vi "Destroy.vi"(8 "error in (no error)":errorcluster, 11 "ServiceName Template in":refnum<class "ServiceName Template.lvclass">) -> (0 "error out":errorcluster, 3 "ServiceName Template out":refnum<class "ServiceName Template.lvclass">)   [LabVIEW 2024, in "ServiceName Template.lvclass"]
uses:
  ServiceName Template.lvclass
  ServiceName Template.lvclass/ServiceName Template.ctl
  gRPC lv Servicer/ServiceBase/ServiceBase.lvclass
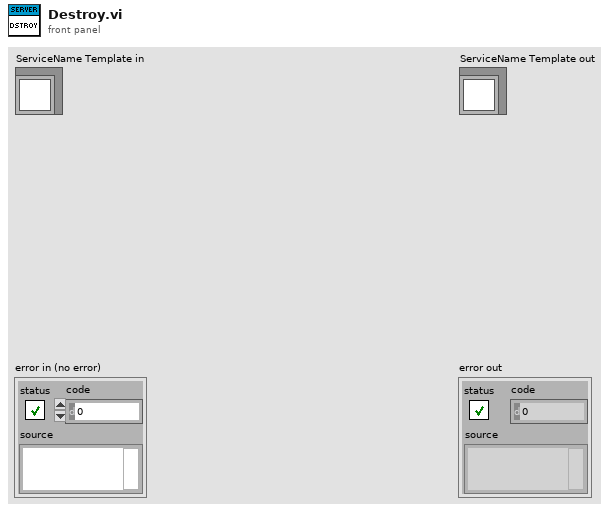
[diagram p1: front panel]
types:
  T1 = typedef "ServiceName Template.lvclass/Server gRPC UEs.ctl" = cluster{"package_service_method":refnum<user-event>}
  T2 = typedef "ServiceName Template.lvclass/Server Internal UEs.ctl" = cluster{"package_service_method Internal UE":refnum<user-event>}
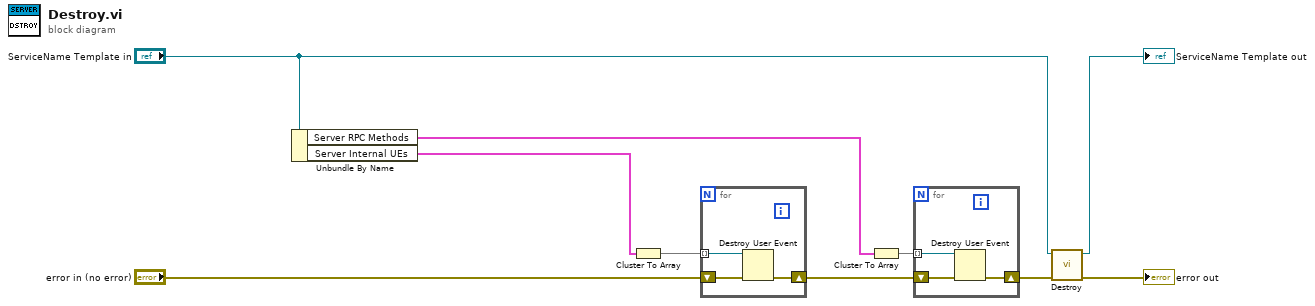
[diagram p0: block diagram]
diagram:
  n1 = Unbundle By Name("ServiceName Template in") -> ("Server RPC Methods"=w4:T1, "Server Internal UEs"=w5:T2)
  n2 = Cluster To Array(cluster=w5) -> (array=w6:refnum<user-event>[])
  n3 = for {
    tunnel: w6 -> [w13] mode=indexing
    shift-right: [w11] -> w2
    shift-left: "error in (no error)" -> [w12]
    n4 = Destroy User Event(user event=w13, error in=w12) -> (error out=w11:errorcluster)
  }
  n5 = Cluster To Array(cluster=w4) -> (array=w3:refnum<user-event>[])
  n6 = for {
    tunnel: w3 -> [w16] mode=indexing
    shift-right: [w14] -> w1
    shift-left: w2 -> [w15]
    n7 = Destroy User Event(user event=w16, error in=w15) -> (error out=w14:errorcluster)
  }
  n8 = call-parent "Destroy.vi"("error in"=w1, "SignalGeneratorService in"="ServiceName Template in") -> ("error out"=→"error out":errorcluster, "SignalGeneratorService out"=→"ServiceName Template out":refnum<class "ServiceName Template.lvclass">)  [unwired: 8 in]
